vi "VannaSelection.vi"(1 "Rotation/position selector: Rot is neg, Pos is positive":dbl, 2 "Vanna Raw throttle (%)":dbl) -> (0 "Vanna Teleop Command":T1)   [LabVIEW 2019]
uses:
  Vanna Command Type Def.ctl
  Vanna Mode Type Def.ctl
panel:
  # "Operator Right joystick X: Vanna Manual. must have deadband.\nOperator Left Joystick Y: UP = Rotation control; DOWN = position control"
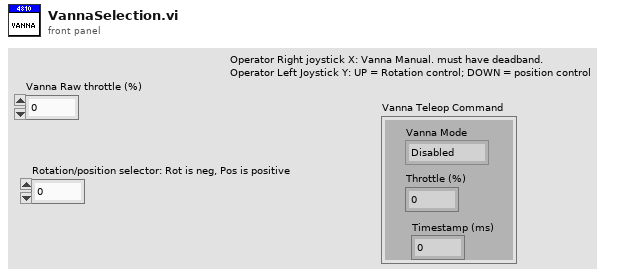
[diagram p1: front panel]
types:
  T1 = typedef "Vanna Command Type Def.ctl" = cluster{"Vanna Mode":T2, "Throttle (%)":dbl, "Timestamp (ms)":dbl}
  T2 = typedef "Vanna Mode Type Def.ctl" = enum16{"Disabled", "Raw Throttle", "Rotation Control", "Position Control"}
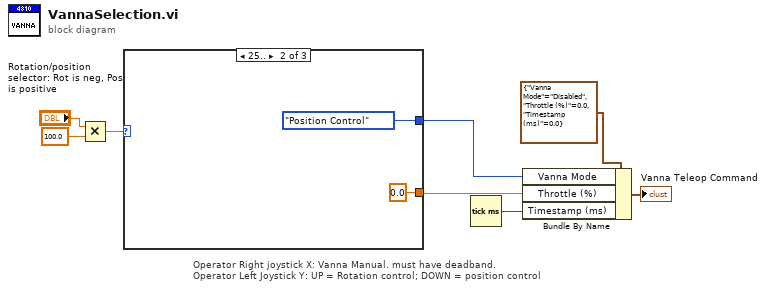
[diagram p0: block diagram]
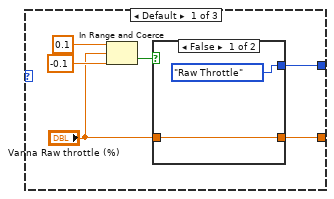
[diagram p2: hidden frame]
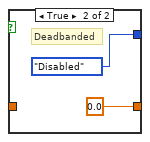
[diagram p3: hidden frame]
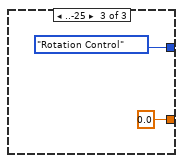
[diagram p4: hidden frame]
diagram:
  # "Operator Right joystick X: Vanna Manual. must have deadband.\nOperator Left Joystick Y: UP = Rotation control; DOWN = position control"
  n1 = Multiply(x="Rotation/position selector: Rot is neg, Pos is positive", y=100.0) -> (x*y=w3:dbl)
  n2 = case shown="25.." w3 {
    tunnel: [w11 Vanna_Mode_Type_Def."Position Control" ("Vanna Mode") Vanna_Mode_Type_Def."Rotation Control" ("Vanna Mode")] -> w2
    tunnel: [w10 0.0 ("Vanna Raw throttle (%)") 0.0 ("Vanna Raw throttle (%)")] -> w1
    frame Default {
      n3 = In Range and Coerce(upper limit=0.1, x="Vanna Raw throttle (%)", lower limit=-0.1 ("upper limit")) -> (In Range?=w12:bool)  [unwired: 1 out]
      n4 = case shown="False" w12 {
        tunnel: [Vanna_Mode_Type_Def."Raw Throttle" ("Vanna Mode") Vanna_Mode_Type_Def."Disabled" ("Vanna Mode")] -> w11
        tunnel: [w15 0.0 ("Vanna Raw throttle (%)")] -> w10
        tunnel: "Vanna Raw throttle (%)" -> [w15 _]
        frame False {
        }
        frame True {
          # "Deadbanded"
        }
      }
    }
    frame 25.. {
    }
    frame ..-25 {
    }
  }
  n5 = Tick Count (ms)() -> (millisecond timer value=w7:u32)
  n6 = Bundle By Name(cluster=T1 {"Vanna Mode"=enum."Disabled", "Throttle (%)"=0.0, "Timestamp (ms)"=0.0} ("Vanna Command"), "Vanna Mode"=w2, "Throttle (%)"=w1, "Timestamp (ms)"=w7) -> (→"Vanna Teleop Command":T1)
